vi "Configure Data Read.vi"(0 "RedPitaya connection in":refnum<k5>, 2 "Read Units":enum16{"", "Raw", "Volts"}(ring), 3 "Data Format":enum16{"", "Binary", "ASCII"}(ring), 5 "error in":errorcluster, 12 "timeout ms (2000)":i32=2000) -> (14 "RedPitaya connection out":refnum<k5>, 19 "error out":errorcluster)   [LabVIEW 2021, in "RedPitaya.lvlib"]
doc: "Confugures units and format in which the acquired data will be returned."
uses:
  RedPitaya.lvlib
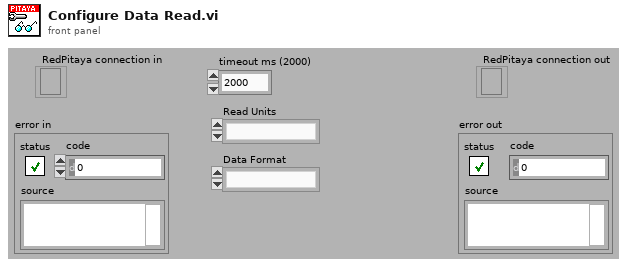
[diagram p1: front panel]
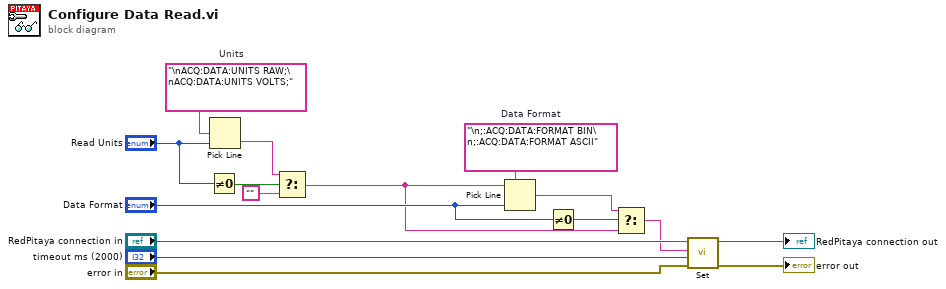
[diagram p0: block diagram]
diagram:
  w6 = "\n;:ACQ:DATA:FORMAT BIN\n;:ACQ:DATA:FORMAT ASCII"  # Data Format
  w10 = "\nACQ:DATA:UNITS RAW;\nACQ:DATA:UNITS VOLTS;"  # Units
  n1 = Not Equal To 0?(x="Read Units") -> (x != 0?=w11:bool)
  n2 = Pick Line(multi-line string=w10, line index="Read Units") -> (output string=w8:string)  [unwired: 1 in]
  n3 = Select(t=w8, s=w11, f="") -> (s? t:f=w2:string)
  n4 = Pick Line(string ("")=w2, multi-line string=w6, line index="Data Format") -> (output string=w5:string)
  n5 = Not Equal To 0?(x="Data Format") -> (x != 0?=w4:bool)
  n6 = Select(t=w5, s=w4, f=w2) -> (s? t:f=w1:string)
  n7 = call "Set.vi"("error in"="error in", "timeout ms (2000)"="timeout ms (2000)", "SCPI Message"=w1, "RedPitaya connection in"="RedPitaya connection in") -> ("error out"=→"error out":errorcluster, "RedPitaya connection out"=→"RedPitaya connection out":refnum<k5>)  [unwired: 5 in, 1 out]
